vi "FPGA_DIOWritePWMValue.vi"(6 "Indicate Zero":bool, 8 "error in (no error)":errorcluster, 9 "PWMValue":u16, 10 "PWMChannel":T2, 11 "DIODeviceRef In":T1) -> (0 "error out":errorcluster, 3 "DIODeviceRef Out":T1)   [LabVIEW 2017]
uses:
  <vilib>/Rock Robotics/SystemInterfaces/DIO/FPGA_DIODevRef.ctl
  <vilib>/Rock Robotics/SystemInterfaces/DIO/FPGA_DIOPWMChannel.ctl
  <vilib>/Rock Robotics/SystemInterfaces/System/FPGA_SystemFPGA Ref Global.vi
  <vilib>/Utility/error.llb/Error Cluster From Error Code.vi
  <vilib>/rvi/errors/niLvFpgaAdjustHostInterfaceError.vi
  <vilib>/rvi/interface/nirviReadWriteControl/nirviReadWriteControl.xnode
  <vilib>/Rock Robotics/SystemInterfaces/System/FPGA_SystemFRC FPGA Ref.ctl
  <vilib>/rvi/interface/Simulation/niFpgaSimulationCallBeginRW.vi
  NiFpgaLv.dll
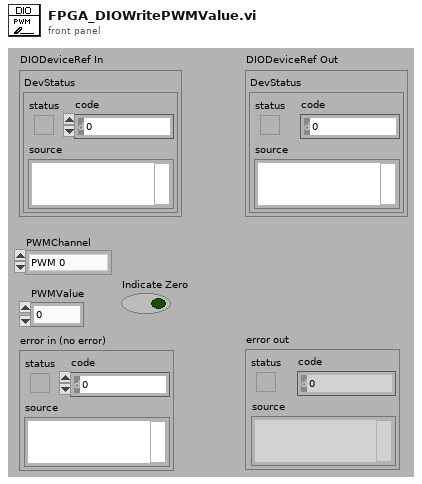
[diagram p1: front panel]
types:
  T1 = typedef "FPGA_DIODevRef.ctl" = cluster{"DevStatus":errorcluster}
  T2 = typedef "FPGA_DIOPWMChannel.ctl" = enum8{"PWM 0", "PWM 1", "PWM 2", "PWM 3", "PWM 4", "PWM 5", "PWM 6", "PWM 7", "PWM 8", "PWM 9", "PWM MXP 0", "PWM MXP 1", "PWM MXP 2", "PWM MXP 3", "PWM MXP 4", "PWM MXP 5", "PWM MXP 6", "PWM MXP 7", "PWM MXP 8", "PWM MXP 9", "Invalid"}
  T3 = typedef "FPGA_SystemFRC FPGA Ref.ctl" = refnum<k20>
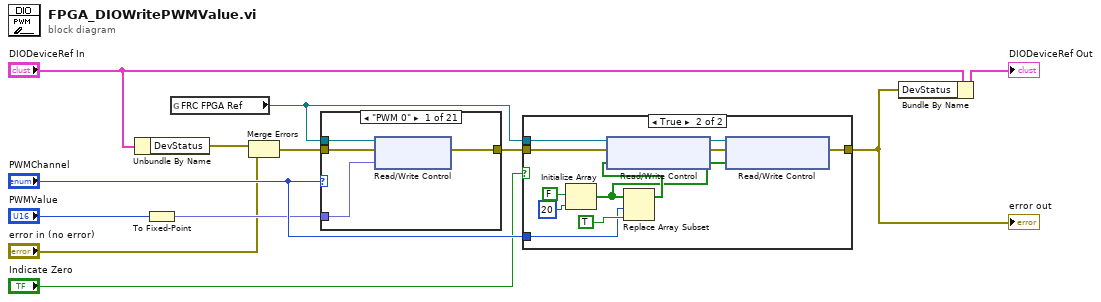
[diagram p0: block diagram]
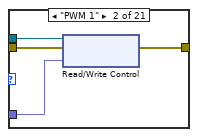
[diagram p3: hidden frame]
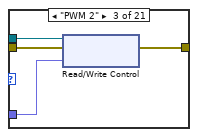
[diagram p4: hidden frame]
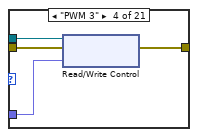
[diagram p5: hidden frame]
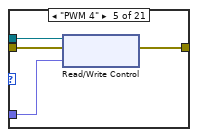
[diagram p6: hidden frame]
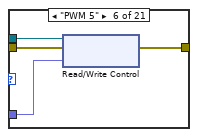
[diagram p7: hidden frame]
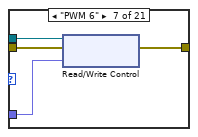
[diagram p8: hidden frame]
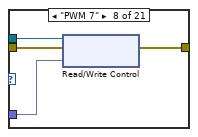
[diagram p9: hidden frame]
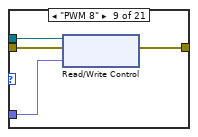
[diagram p10: hidden frame]
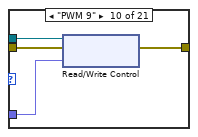
[diagram p11: hidden frame]
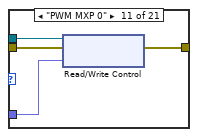
[diagram p12: hidden frame]
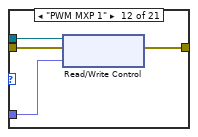
[diagram p13: hidden frame]
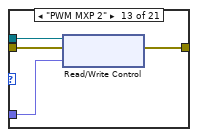
[diagram p14: hidden frame]
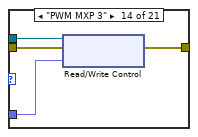
[diagram p15: hidden frame]
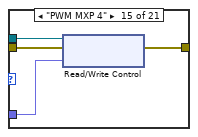
[diagram p16: hidden frame]
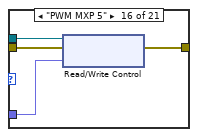
[diagram p17: hidden frame]
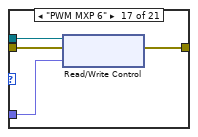
[diagram p18: hidden frame]
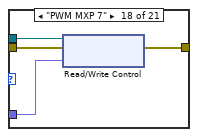
[diagram p19: hidden frame]
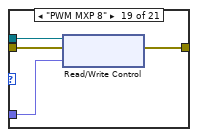
[diagram p20: hidden frame]
diagram:
  n1 = Unbundle By Name("DIODeviceRef In") -> ("DevStatus"=w7:errorcluster)
  n2 = To Fixed-Point(number="PWMValue") -> (fixed-point=w5:fxp<+,12,12>)  [unwired: 1 in]
  n3 = global read "FPGA_SystemFPGA Ref Global.vi" "FRC FPGA Ref"() -> (w8:T3)
  n4 = Merge Errors(w7, "error in (no error)") -> (w6:errorcluster)
  n5 = case shown="\"PWM 0\"" "PWMChannel" {
    tunnel: w8 -> [w16 w17 w21 w25 w29 w33 w37 w41 w46 w49 w56 w60 w64 w68 w72 w76 w80 w84 w88 w92 _]
    tunnel: w6 -> [w15 w18 w22 w26 w30 w34 w38 w42 w45 w50 w55 w57 w63 w67 w71 w75 w79 w83 w87 w91 w94]
    tunnel: [w13 w19 w23 w27 w31 w35 w39 w43 w47 w51 w54 w58 w62 w66 w70 w74 w78 w82 w86 w90 w93] -> w3
    tunnel: w5 -> [w14 w20 w24 w28 w32 w36 w40 w44 w48 w52 w53 w59 w61 w65 w69 w73 w77 w81 w85 w89 _]
    frame "PWM 0" {
      n6 = xnode "Read/Write Control"("FPGA VI Reference In"=w16, "error in"=w15, "PWM.Hdr0"=w14) -> ("error out"=w13:errorcluster)  [unwired: 1 out]
    }
    frame "PWM 1" {
      n7 = xnode "Read/Write Control"("FPGA VI Reference In"=w17, "error in"=w18, "PWM.Hdr1"=w20) -> ("error out"=w19:errorcluster)  [unwired: 1 out]
    }
    frame "PWM 2" {
      n8 = xnode "Read/Write Control"("FPGA VI Reference In"=w21, "error in"=w22, "PWM.Hdr2"=w24) -> ("error out"=w23:errorcluster)  [unwired: 1 out]
    }
    frame "PWM 3" {
      n9 = xnode "Read/Write Control"("FPGA VI Reference In"=w25, "error in"=w26, "PWM.Hdr3"=w28) -> ("error out"=w27:errorcluster)  [unwired: 1 out]
    }
    frame "PWM 4" {
      n10 = xnode "Read/Write Control"("FPGA VI Reference In"=w29, "error in"=w30, "PWM.Hdr4"=w32) -> ("error out"=w31:errorcluster)  [unwired: 1 out]
    }
    frame "PWM 5" {
      n11 = xnode "Read/Write Control"("FPGA VI Reference In"=w33, "error in"=w34, "PWM.Hdr5"=w36) -> ("error out"=w35:errorcluster)  [unwired: 1 out]
    }
    frame "PWM 6" {
      n12 = xnode "Read/Write Control"("FPGA VI Reference In"=w37, "error in"=w38, "PWM.Hdr6"=w40) -> ("error out"=w39:errorcluster)  [unwired: 1 out]
    }
    frame "PWM 7" {
      n13 = xnode "Read/Write Control"("FPGA VI Reference In"=w41, "error in"=w42, "PWM.Hdr7"=w44) -> ("error out"=w43:errorcluster)  [unwired: 1 out]
    }
    frame "PWM 8" {
      n14 = xnode "Read/Write Control"("FPGA VI Reference In"=w46, "error in"=w45, "PWM.Hdr8"=w48) -> ("error out"=w47:errorcluster)  [unwired: 1 out]
    }
    frame "PWM 9" {
      n15 = xnode "Read/Write Control"("FPGA VI Reference In"=w49, "error in"=w50, "PWM.Hdr9"=w52) -> ("error out"=w51:errorcluster)  [unwired: 1 out]
    }
    frame "PWM MXP 0" {
      n16 = xnode "Read/Write Control"("FPGA VI Reference In"=w56, "error in"=w55, "PWM.MXP0"=w53) -> ("error out"=w54:errorcluster)  [unwired: 1 out]
    }
    frame "PWM MXP 1" {
      n17 = xnode "Read/Write Control"("FPGA VI Reference In"=w60, "error in"=w57, "PWM.MXP1"=w59) -> ("error out"=w58:errorcluster)  [unwired: 1 out]
    }
    frame "PWM MXP 2" {
      n18 = xnode "Read/Write Control"("FPGA VI Reference In"=w64, "error in"=w63, "PWM.MXP2"=w61) -> ("error out"=w62:errorcluster)  [unwired: 1 out]
    }
    frame "PWM MXP 3" {
      n19 = xnode "Read/Write Control"("FPGA VI Reference In"=w68, "error in"=w67, "PWM.MXP3"=w65) -> ("error out"=w66:errorcluster)  [unwired: 1 out]
    }
    frame "PWM MXP 4" {
      n20 = xnode "Read/Write Control"("FPGA VI Reference In"=w72, "error in"=w71, "PWM.MXP4"=w69) -> ("error out"=w70:errorcluster)  [unwired: 1 out]
    }
    frame "PWM MXP 5" {
      n21 = xnode "Read/Write Control"("FPGA VI Reference In"=w76, "error in"=w75, "PWM.MXP5"=w73) -> ("error out"=w74:errorcluster)  [unwired: 1 out]
    }
    frame "PWM MXP 6" {
      n22 = xnode "Read/Write Control"("FPGA VI Reference In"=w80, "error in"=w79, "PWM.MXP6"=w77) -> ("error out"=w78:errorcluster)  [unwired: 1 out]
    }
    frame "PWM MXP 7" {
      n23 = xnode "Read/Write Control"("FPGA VI Reference In"=w84, "error in"=w83, "PWM.MXP7"=w81) -> ("error out"=w82:errorcluster)  [unwired: 1 out]
    }
    frame "PWM MXP 8" {
      n24 = xnode "Read/Write Control"("FPGA VI Reference In"=w88, "error in"=w87, "PWM.MXP8"=w85) -> ("error out"=w86:errorcluster)  [unwired: 1 out]
    }
    frame "PWM MXP 9" {
      n25 = xnode "Read/Write Control"("FPGA VI Reference In"=w92, "error in"=w91, "PWM.MXP9"=w89) -> ("error out"=w90:errorcluster)  [unwired: 1 out]
    }
    frame "Invalid" {
      n26 = call <vilib>:"FPGA_DIOERRInvalidPWMChannel.vi"("error in (no error)"=w94) -> ("error out"=w93:errorcluster)
    }
  }
  n27 = case shown="True" "Indicate Zero" {
    tunnel: w3 -> [w95 w106]
    tunnel: w8 -> [_ w105]
    tunnel: [w95 w102] -> w9
    tunnel: "PWMChannel" -> [_ w98]
    frame False {
    }
    frame True {
      n28 = Initialize Array(FALSE, 20 ("dimension size")) -> (w96:bool[])
      n29 = Replace Array Subset(array=w96, new element=TRUE, index=w98) -> (w97:bool[])
      n30 = xnode "Read/Write Control"("FPGA VI Reference In"=w105, "error in"=w106, "PWM.ZeroLatch"=w97) -> ("FPGA VI Reference Out"=w100:T3, "error out"=w101:errorcluster)
      n31 = xnode "Read/Write Control"("FPGA VI Reference In"=w100, "error in"=w101, "PWM.ZeroLatch"=w96) -> ("error out"=w102:errorcluster)  [unwired: 1 out]
    }
  }
  "error out" <- w9
  n32 = Bundle By Name(cluster="DIODeviceRef In", "DevStatus"=w9) -> (→"DIODeviceRef Out":T1)
